vi "CSTK_MCListbox_Designer_MoveDownColHdr.vi"(7 "表头属性列表输入":refnum<vi>, 8 "错误输入（无错误）":errorcluster, 9 "Selected Index":i32, 10 "MCListbox引用句柄":refnum<vi>, 11 "VI输入":refnum<vi>) -> (0 "错误输出":errorcluster, 3 "VI输出":refnum<vi>)   [LabVIEW 2015, in "CSTK_MCListbox Designer.lvlib"]
uses:
  CSTK_MCListbox Designer.lvlib
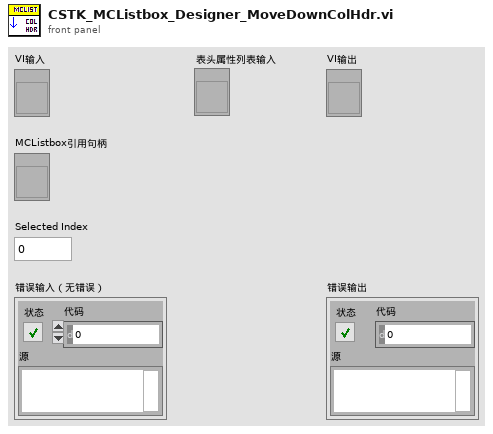
[diagram p1: front panel]
types:
  T1 = typedef "CSTK_MCListbox Designer.lvlib/_CSTK_MCListbox_Designer_ColHdr_Selected.ctl" = cluster{"选择":bool, "表头属性":T2}
  T2 = typedef "CSTK_MCListbox Designer.lvlib/_CSTK_MCListbox_Designer_ColHdr.ctl" = cluster{"列名称":string, "单元格宽度":u32, "粗体":bool, "斜体":bool, "对齐":enum16{"Left", "Center", "Right"}}
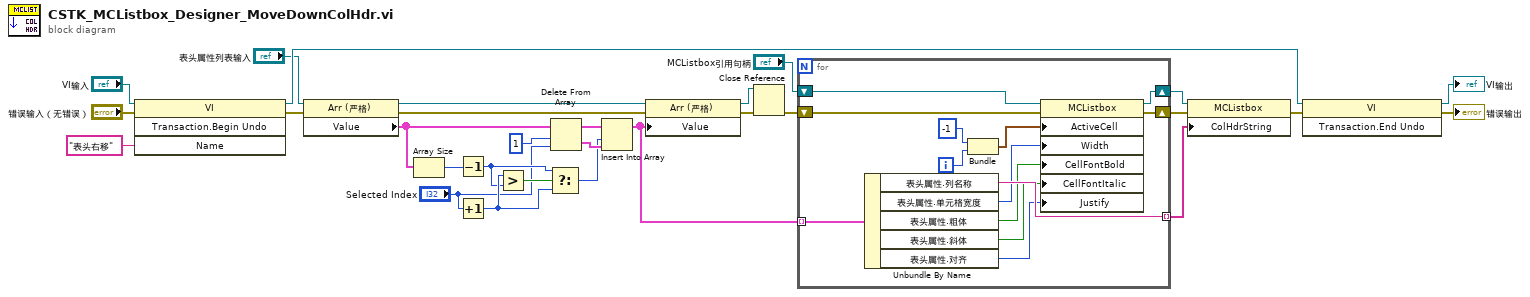
[diagram p0: block diagram]
diagram:
  n1 = invoke class="VI" method="Transaction.Begin Undo"(reference="VI输入", error in="错误输入（无错误）", "Name"="表头右移" ("名称")) -> (reference out=w17:refnum<vi>, error out=w25:errorcluster)  [unwired: 1 in, 2 out]
  n2 = property on="属性节点" class="Arr (严格)"(reference="表头属性列表输入", error in=w25) -> (reference out=w13:refnum<vi>, error out=w11:errorcluster, "Value"=w4:T1[])
  n3 = Array Size(array=w4) -> (size(s)=w8:i32)
  n4 = Decrement(x=w8) -> (x-1=w6:i32)
  n5 = Increment(x="Selected Index") -> (x+1=w7:i32)
  n6 = Greater?(x=w7, y=w6) -> (0:w5:bool)
  n7 = Select(t=w6, s=w5, f=w7) -> (s? t:f=w3:i32)
  n8 = Delete From Array(array=w4, length=1 ("长度"), index="Selected Index") -> (deleted portion=w14:T1[], array with subset deleted=w15:T1[])
  n9 = Insert Into Array(array=w15, index=w3, new element=w14) -> (w10:T1[])
  n10 = property on="属性节点" class="Arr (严格)"(reference=w13, error in=w11, "Value"=w10) -> (reference out=w12:refnum<vi>, error out=w9:errorcluster)
  n11 = Close Reference(reference=w12, error in (no error)=w9) -> (error out=w16:errorcluster)
  n12 = for {
    tunnel: w10 -> [w40] mode=indexing
    tunnel: [w39] -> w28 mode=indexing
    shift-right: [w36] -> w26
    shift-left: "MCListbox引用句柄" -> [w37]
    shift-right: [w31] -> w27
    shift-left: w16 -> [w32]
    i -> [w41]
    n13 = Unbundle By Name(w40) -> ("表头属性.列名称"=w39:string, "表头属性.单元格宽度"=w35:u32, "表头属性.粗体"=w34:bool, "表头属性.斜体"=w30:bool, "表头属性.对齐"=w33:enum16{"Left", "Center", "Right"})
    n14 = Bundle(-1, w41) -> (w38:cluster{i32, i32})  [unwired: 1 in]
    n15 = property class="MCListbox"(reference=w37, error in=w32, "ActiveCell"=w38, "Width"=w35, "CellFontBold"=w34, "CellFontItalic"=w30, "Justify"=w33) -> (reference out=w36:refnum<vi>, error out=w31:errorcluster)
  }
  n16 = property class="MCListbox"(reference=w26, error in=w27, "ColHdrString"=w28) -> (error out=w29:errorcluster)  [unwired: 1 out]
  n17 = invoke class="VI" method="Transaction.End Undo"(reference=w17, error in=w29) -> (reference out=→"VI输出":refnum<vi>, error out=→"错误输出":errorcluster)  [unwired: 1 in, 1 out]
